vi "Mostrar_nombres_obtener_path HOCG.vi"(6 "Cancion actual":u32, 9 "Lista actual":u32, 10 "folder names":string[](array[string]), 11 "path in":path) -> (0 "Lista actual":string, 1 "Artista":string, 2 "Lista":string[](array[string]), 3 "Path de cancion":path, 4 "Canción":string, 5 "Cantidad de canciones":i32)   [LabVIEW 2021]
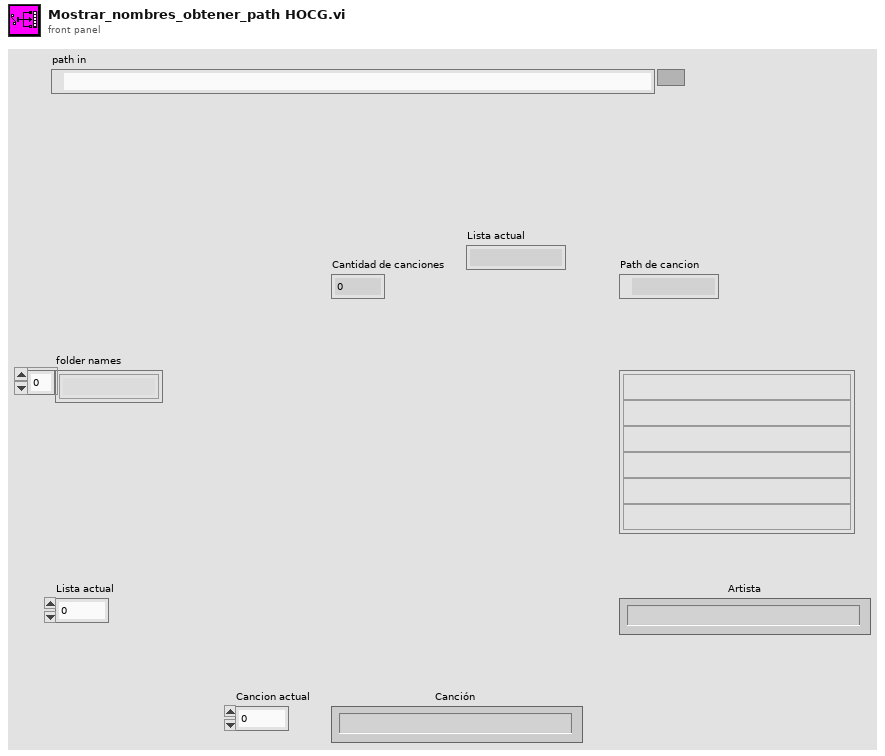
[diagram p1: front panel]
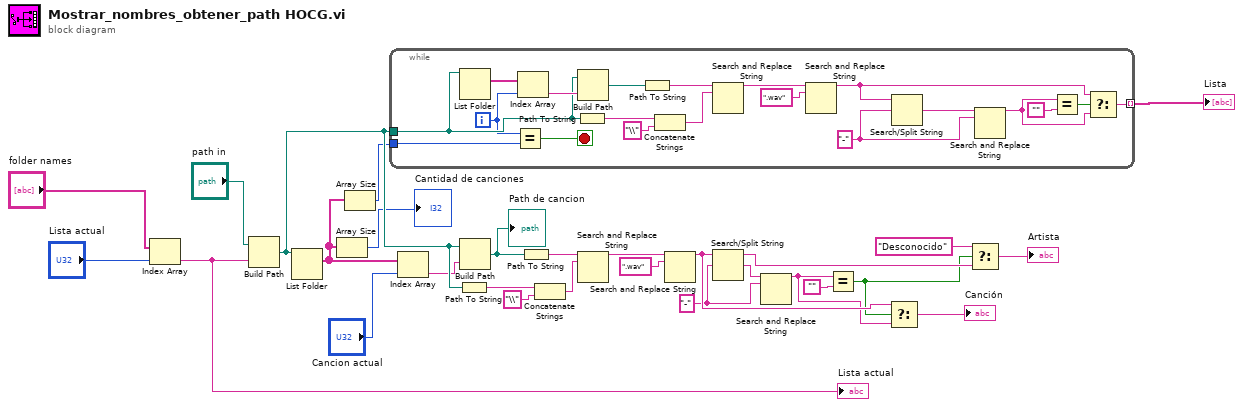
[diagram p0: block diagram]
diagram:
  w7 = "-" ("search string/char (-)")
  n1 = Index Array(array="folder names", index="Lista actual") -> (element=w1:string)
  "Lista actual" <- w1
  n2 = Build Path(base path="path in", name or relative path=w1) -> (appended path=w28:path)
  n3 = List Folder(path=w28) -> (filenames=w9:string[])  [unwired: 3 in, 3 out]
  n4 = Array Size(array=w9) -> (size(s)=→"Cantidad de canciones":i32)
  n5 = Array Size(array=w9) -> (size(s)=w10:i32)
  n6 = while {
    tunnel: [w29] -> w3 mode=indexing
    tunnel: w10 -> [w44]
    tunnel: w28 -> [w35]
    i -> [w34]
    stop <- w47 stop-if-true
    w46 = "-" ("search string/char (-)")
    n7 = List Folder(path=w35) -> (filenames=w38:string[])  [unwired: 3 in, 3 out]
    n8 = Equal?(x=w34, y=w44) -> (x = y?=w47:bool)
    n9 = Index Array(array=w38, index=w34) -> (element=w37:string)
    n10 = Path To String(path=w35) -> (string=w42:string)
    n11 = Build Path(base path=w35, name or relative path=w37) -> (appended path=w36:path)
    n12 = Path To String(path=w36) -> (string=w43:string)
    n13 = Concatenate Strings(w42, "\\" ("string")) -> (w40:string)
    n14 = Search and Replace String(input string=w43, search string=w40) -> (result string=w39:string)  [unwired: 6 in, 3 out]
    n15 = Search and Replace String(input string=w39, search string=".wav") -> (result string=w30:string)  [unwired: 6 in, 3 out]
    n16 = Search/Split String(string=w30, search string/char (-)=w46) -> (match + rest of string=w45:string)  [unwired: 1 in, 2 out]
    n17 = Search and Replace String(input string=w45, search string=w46) -> (result string=w31:string)  [unwired: 6 in, 3 out]
    n18 = Equal?(x=w31, y="") -> (x = y?=w32:bool)
    n19 = Select(t=w30, s=w32, f=w31) -> (s? t:f=w29:string)
  }
  "Lista" <- w3
  n20 = Index Array(array=w9, index="Cancion actual") -> (element=w5:string)
  n21 = Path To String(path=w28) -> (string=w22:string)
  n22 = Build Path(base path=w28, name or relative path=w5) -> (appended path=w27:path)
  "Path de cancion" <- w27
  n23 = Path To String(path=w27) -> (string=w21:string)
  n24 = Concatenate Strings(w22, "\\" ("string")) -> (w24:string)
  n25 = Search and Replace String(input string=w21, search string=w24) -> (result string=w25:string)  [unwired: 6 in, 3 out]
  n26 = Search and Replace String(input string=w25, search string=".wav") -> (result string=w26:string)  [unwired: 6 in, 3 out]
  n27 = Search/Split String(string=w26, search string/char (-)=w7) -> (substring before match=w17:string, match + rest of string=w8:string)  [unwired: 1 in, 1 out]
  n28 = Search and Replace String(input string=w8, search string=w7) -> (result string=w18:string)  [unwired: 6 in, 3 out]
  n29 = Equal?(x=w18, y="") -> (x = y?=w16:bool)
  n30 = Select(t=w26, s=w16, f=w18) -> (s? t:f=→"Canción":string)
  n31 = Select(t="Desconocido", s=w16, f=w17) -> (s? t:f=→"Artista":string)
